vi "GetTaskBarItemNamesUser32DLL.vi"() -> ()   [LabVIEW 2014]
uses:
  C:/Windows/System32/user32.dll
panel:
  out "hToolbar 2":u32
  out "hTask":u32
  out "hToolbar":u32
  out "hReBar":u32
  out "hTray":u32
  out "hDesktop":u32
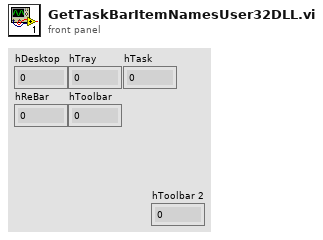
[diagram p1: front panel]
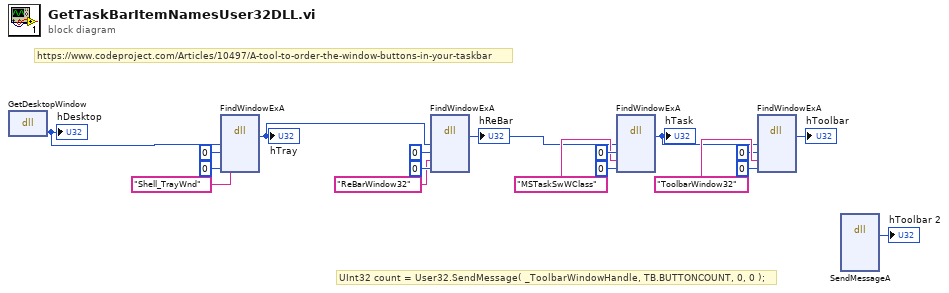
[diagram p0: block diagram]
diagram:
  # "UInt32 count = User32.SendMessage( _ToolbarWindowHandle, TB.BUTTONCOUNT, 0, 0 );"
  # "https://www.codeproject.com/Articles/10497/A-tool-to-order-the-window-buttons-in-your-taskbar"
  n1 = dll-call lib="C:/Windows/System32/user32.dll" fn="GetDesktopWindow"() -> ("hDesktop"=w18:u32)  [unwired: 3 in, 2 out]
  "hDesktop" <- w18
  n2 = dll-call lib="C:/Windows/System32/user32.dll" fn="FindWindowExA"("hwndParent"=w18, "hwndChildAfter"=u32 0, "lpszClass"="Shell_TrayWnd", "lpszWindow"=u32 0) -> ("hTray"=w14:u32)  [unwired: 7 in, 2 out]
  "hTray" <- w14
  n3 = dll-call lib="C:/Windows/System32/user32.dll" fn="FindWindowExA"("hwndParent"=w14, "hwndChildAfter"=u32 0, "lpszClass"="ReBarWindow32", "lpszWindow"=u32 0) -> ("hReBar"=w7:u32)  [unwired: 7 in, 2 out]
  "hReBar" <- w7
  n4 = dll-call lib="C:/Windows/System32/user32.dll" fn="FindWindowExA"("hwndParent"=w7, "hwndChildAfter"=u32 0, "lpszClass"="MSTaskSwWClass", "lpszWindow"=u32 0) -> ("hTask"=w3:u32)  [unwired: 7 in, 2 out]
  "hTask" <- w3
  n5 = dll-call lib="C:/Windows/System32/user32.dll" fn="FindWindowExA"("hwndParent"=w3, "hwndChildAfter"=u32 0, "lpszClass"="ToolbarWindow32", "lpszWindow"=u32 0) -> ("hToolbar"=→"hToolbar":u32)  [unwired: 7 in, 2 out]
  n6 = dll-call lib="C:/Windows/System32/user32.dll" fn="SendMessageA"() -> ("hToolbar"=→"hToolbar 2":u32)  [unwired: 11 in, 2 out]
